vi "MB Serial String to Modbus Data Unit.vi"(7 "Mode":enum16{"RTU", "ASCII"}(ring), 8 "error in (no error)":errorcluster, 11 "String":string) -> (0 "error out":errorcluster, 1 "Exception Code":u8 format="%.0x", 2 "Slave Address":u8 format="%.0x", 3 "Modbus Data Unit":T1={"Function Code"=1, "Data"=[]} {"Function Code" items=["Read Coils"=1, "Read Discrete Inputs"=2, "Read Holding Registers"=3, "Read Input Registers"=4, "Write Single Coil"=5, "Write Single Register"=6, "Read Exception Status"=7, "Write Multiple Coils"=15, "Write Multiple Registers"=16]; "Data" format="%.0x"})   [LabVIEW 2012]
uses:
  MB Modbus Data Unit.ctl
panel:
  # "VI Name: MB Serial String to Modbus Data Unit.vi\nPurpose: Formats the string received in a Modbus Data Unit.\nReentrant VI, because its caller is also reentrant."
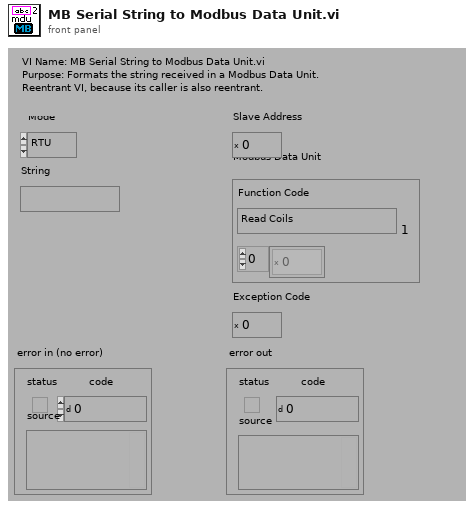
[diagram p1: front panel]
types:
  T1 = typedef "MB Modbus Data Unit.ctl" = cluster{"Function Code":u8, "Data":u8[]}
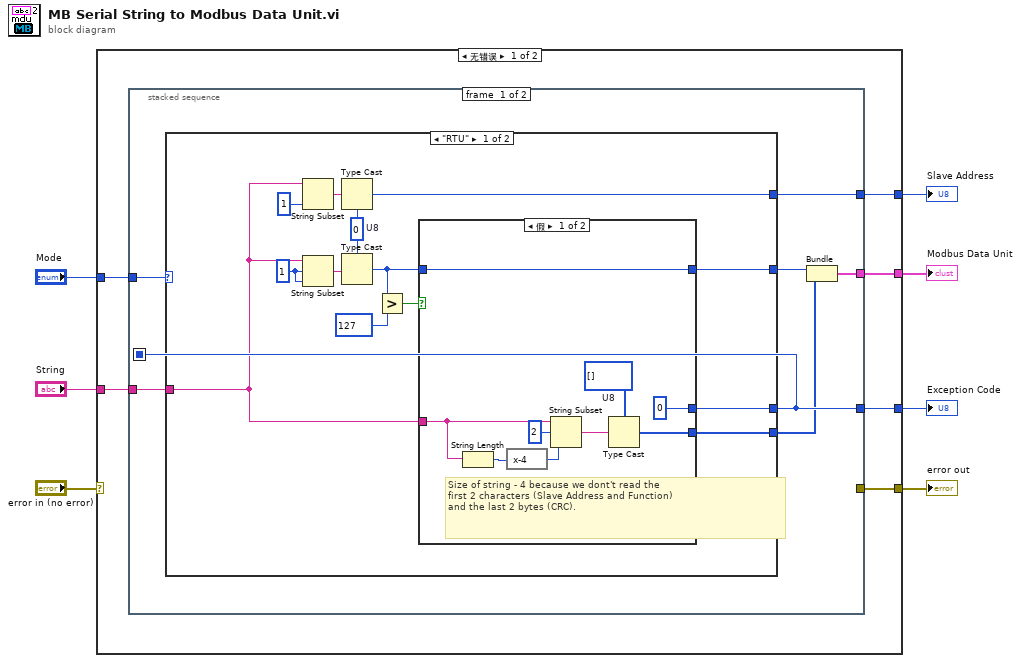
[diagram p0: block diagram]
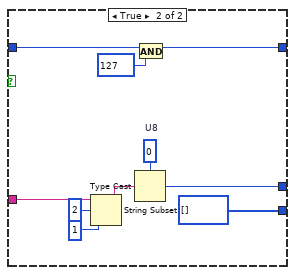
[diagram p2: hidden frame]
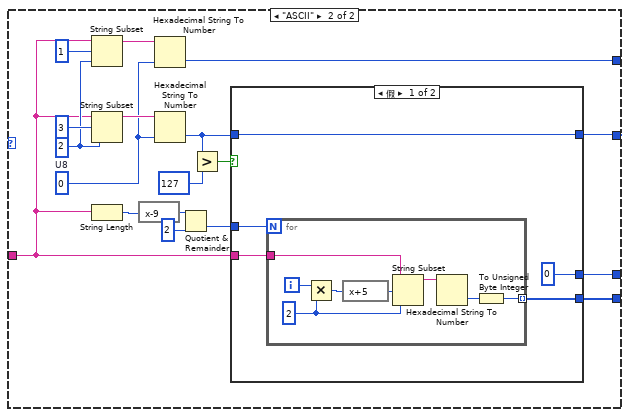
[diagram p3: hidden frame]
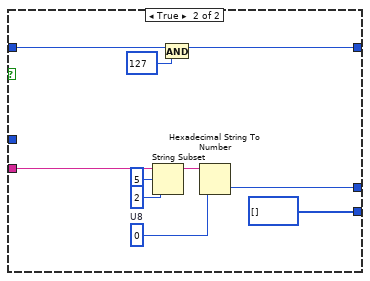
[diagram p4: hidden frame]
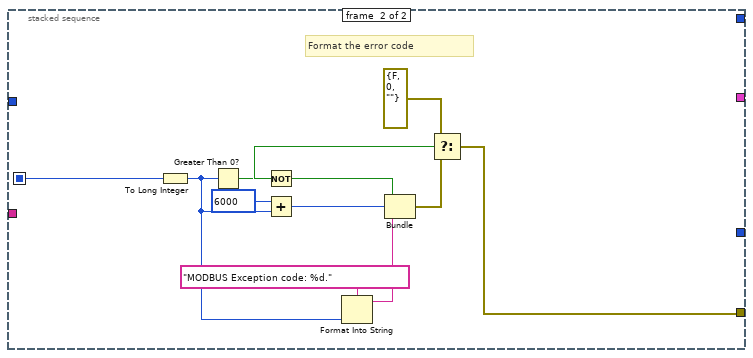
[diagram p5: hidden frame]
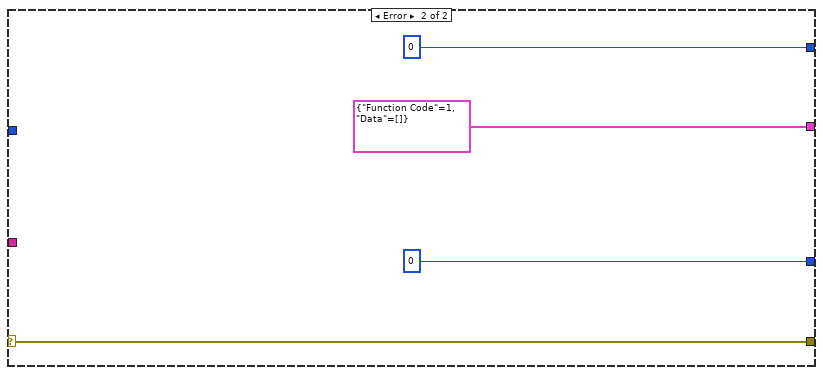
[diagram p6: hidden frame]
diagram:
  n1 = case shown="无错误" "error in (no error)" {
    selector: "error in (no error)" -> [_ w108]
    tunnel: "String" -> [w13 _]
    tunnel: "Mode" -> [w12 _]
    tunnel: [w11 u8 0 ("U8")] -> w5
    tunnel: [w10 w108] -> w3
    tunnel: [w9 T1 {"Function Code"=1, "Data"=[]} ("MODBUS Data Unit")] -> w2
    tunnel: [w8 u8 0] -> w1
    frame No Error {
      n2 = stacked-sequence {
        seq-local: [w18 _] -> [_ w98]
        tunnel: w13 -> [w20 _]
        tunnel: w12 -> [w19 _]
        tunnel: [w18 _] -> w11
        tunnel: [_ w97] -> w10
        tunnel: [w15 _] -> w9
        tunnel: [w14 _] -> w8
        frame #0 {
          n3 = case shown="\"RTU\"" w19 {
            tunnel: w20 -> [w22 w53]
            tunnel: [w26 w63] -> w17
            tunnel: [w23 w62] -> w16
            tunnel: [w29 w60] -> w14
            tunnel: [w25 w59] -> w18
            frame "RTU" {
              w30 = u8 0  # U8
              w21 = 1
              n4 = String Subset(string=w22, length (rest)=1) -> (substring=w32:string)  [unwired: 1 out]
              n5 = String Subset(string=w22, offset (0)=w21, length (rest)=w21) -> (substring=w31:string)
              n6 = Type Cast(type=w30, x=w32) -> (*(type *) &x=w29:u8)
              n7 = Type Cast(type=w30, x=w31) -> (*(type *) &x=w24:u8)
              n8 = Greater?(x=w24, y=u8 127) -> (0:w27:bool)
              n9 = case shown="假" w27 {
                tunnel: w22 -> [w41 w47]
                tunnel: [w39 u8[] [] ("U8")] -> w26
                tunnel: [u8 0 w46] -> w25
                tunnel: w24 -> [w37 w51]
                tunnel: [w37 w50] -> w23
                frame False {
                  w36 = u8[] []  # U8
                  # "Size of string - 4 because we dont't read the\nfirst 2 characters (Slave Address and Function)\nand the last 2 bytes (CRC)."
                  n10 = String Length(string=w41) -> (length=w35:i32)
                  n11 = expression code="x-4"(w35) -> (w34:i32)
                  n12 = String Subset(string=w41, offset (0)=2, length (rest)=w34) -> (substring=w40:string)
                  n13 = Type Cast(type=w36, x=w40) -> (*(type *) &x=w39:u8[])
                }
                frame True {
                  w49 = u8 0  # U8
                  n14 = String Subset(string=w47, offset (0)=2, length (rest)=1) -> (substring=w48:string)
                  n15 = Type Cast(type=w49, x=w48) -> (*(type *) &x=w46:u8)
                  n16 = And(x=w51, y=u8 127) -> (x .and. y?=w50:u8)
                }
              }
            }
            frame "ASCII" {
              w66 = u8 0  # U8
              w58 = 2
              n17 = String Subset(string=w53, offset (0)=1, length (rest)=w58) -> (substring=w68:string)
              n18 = String Subset(string=w53, offset (0)=3, length (rest)=w58) -> (substring=w67:string)
              n19 = String Length(string=w53) -> (length=w56:i32)
              n20 = expression code="x-9"(w56) -> (w57:i32)
              n21 = Hexadecimal String To Number(string=w68, default (0uL)=w66) -> (number=w60:u8)  [unwired: 2 out]
              n22 = Hexadecimal String To Number(string=w67, default (0uL)=w66) -> (number=w61:u8)  [unwired: 2 out]
              n23 = Quotient & Remainder(x=w57, y=2) -> (floor(x/y)=w54:i32)  [unwired: 1 out]
              n24 = Greater?(x=w61, y=u8 127) -> (0:w64:bool)
              n25 = case shown="假" w64 {
                tunnel: w53 -> [w74 w88]
                tunnel: [w75 u8[] [] ("U8")] -> w63
                tunnel: [w73 w85] -> w62
                tunnel: w61 -> [w73 w93]
                tunnel: [u8 0 w86] -> w59
                tunnel: w54 -> [w71 _]
                frame False {
                  n26 = for {
                    N: w71 -> [_]
                    tunnel: w74 -> [w82]
                    tunnel: [w80] -> w75 mode=indexing
                    i -> [w79]
                    w78 = 2
                    n27 = Multiply(x=w79, y=w78) -> (x*y=w77:i32)
                    n28 = expression code="x+5"(w77) -> (w76:i32)
                    n29 = String Subset(string=w82, offset (0)=w76, length (rest)=w78) -> (substring=w83:string)
                    n30 = Hexadecimal String To Number(string=w83) -> (number=w81:u32)  [unwired: 3 out]
                    n31 = To Unsigned Byte Integer(number=w81) -> (unsigned 8bit integer=w80:u8)
                  }
                }
                frame True {
                  w87 = u8 0  # U8
                  n32 = String Subset(string=w88, offset (0)=5, length (rest)=2) -> (substring=w89:string)
                  n33 = And(x=w93, y=u8 127) -> (x .and. y?=w85:u8)
                  n34 = Hexadecimal String To Number(string=w89, default (0uL)=w87) -> (number=w86:u8)  [unwired: 2 out]
                }
              }
            }
          }
          n35 = Bundle("U8"=w16, "U8"=w17) -> (w15:cluster{"U8":u8, "U8":u8[]})  [unwired: 1 out]
        }
        frame #1 {
          # "Format the error code"
          n36 = To Long Integer(number=w98) -> (32bit integer=w94:i32)
          n37 = Greater Than 0?(x=w94) -> (x > 0?=w101:bool)
          n38 = Not(x=w101) -> (.not. x?=w102:bool)
          n39 = Add(x=6000 ("New Error Code"), y=w94) -> (x+y=w96:i32)
          n40 = Format Into String(format string="MODBUS Exception code: %d.", w94) -> (resulting string=w100:string)  [unwired: 2 in, 1 out]
          n41 = Bundle(w101, w96, w100) -> (w103:errorcluster)  [unwired: 1 out]
          n42 = Select(t=errorcluster {"status"=FALSE, "code"=0, "source"=""} ("error out"), s=w102, f=w103) -> (s? t:f=w97:errorcluster)
        }
      }
    }
    frame Error {
    }
  }
  "error out" <- w3
  "Exception Code" <- w5
  "Modbus Data Unit" <- w2
  "Slave Address" <- w1
